vi "Replace Column Object.vi"(8 "error in (no error)":errorcluster, 10 "Column Object":refnum<class "Column Interface.lvclass">, 11 "Table in":refnum<class "Table.lvclass">) -> (0 "error out":errorcluster, 3 "Table out":refnum<class "Table.lvclass">)   [LabVIEW 2020, in "Table.lvlib" / "Table.lvclass"]
uses:
  Table.lvclass
  Column Interface/Column Interface Class/Column Interface.lvclass
  Table.lvclass/Table.ctl
  <vilib>/Utility/miscctls.llb/LVMapReplaceAction.ctl
  Table Configuration Interface/Table Configuration Interface.lvclass
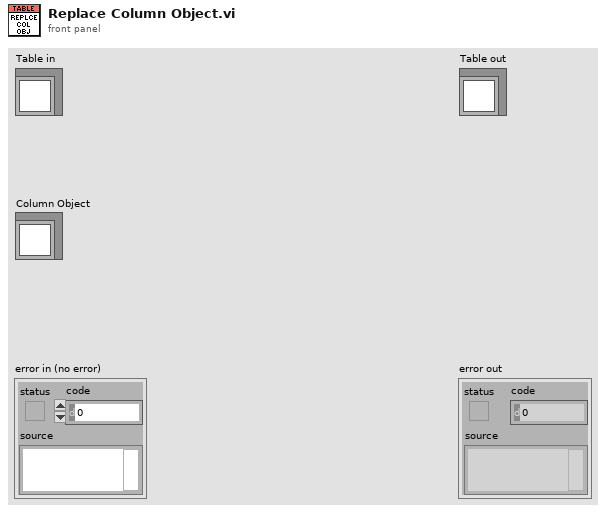
[diagram p1: front panel]
types:
  T1 = typedef "LVMapReplaceAction.ctl" = enum32{"Modify Entry only if found", "Add or Modify Entry", "Delete Entry"}
  T2 = map{string, refnum<class "Column Interface.lvclass">}
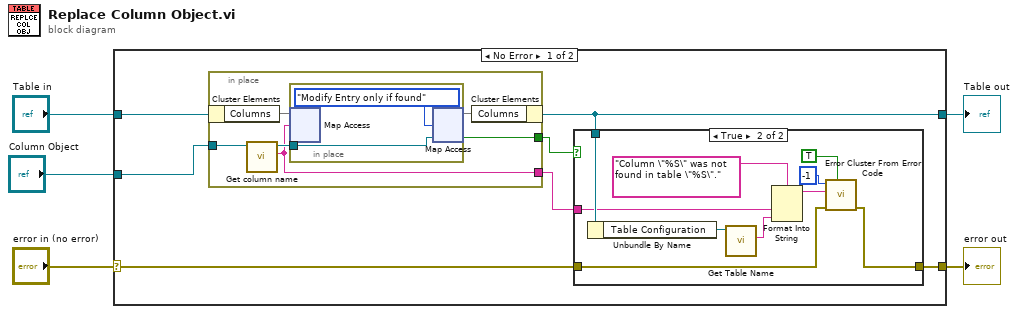
[diagram p0: block diagram]
diagram:
  n1 = case shown="No Error" "error in (no error)" {
    selector: "error in (no error)" -> [w6 w33]
    tunnel: [w7 w33] -> w4
    tunnel: [w10 w32] -> w2
    tunnel: "Table in" -> [w12 w32]
    tunnel: "Column Object" -> [w11 _]
    frame No Error {
      n2 = in-place {
        in-place-border: w11 -> [w29]
        in-place-border: [w25] -> w9
        in-place-border: [w24] -> w8
        n3 = in-place-cluster #1(w12) -> ("Columns"=w28:T2)
        n4 = call-dynamic "Get column name.vi"("Column Interface in"=w29) -> ("Name"=w24:string, "Column Interface out"=w27:refnum<class "Column Interface.lvclass">)  [unwired: 8 in, 1 out]
        n5 = in-place {
          in-place-border: w27 -> [w30]
          n6 = in-place-map #2(w28, w24) -> ()  [unwired: 1 in, 2 out]
          n7 = in-place-map #2(w30, LVMapReplaceAction."Modify Entry only if found" ("action")) -> (w26:T2, w25:bool)  [unwired: 1 out]
        }
        n8 = in-place-cluster #1("Columns"=w26) -> (w10:refnum<class "Table.lvclass">)
      }
      n9 = case shown="True" w9 {
        tunnel: w10 -> [_ w22]
        tunnel: w8 -> [_ w20]
        tunnel: [w13 w15] -> w7
        tunnel: w6 -> [w13 w14]
        frame False {
        }
        frame True {
          n10 = Unbundle By Name(w22) -> ("Table Configuration"=w21:refnum<class "Table Configuration Interface.lvclass">)
          n11 = call-dynamic "Get Table Name.vi"("Table Configuration Interface in"=w21) -> ("Table Name"=w19:string)  [unwired: 8 in, 2 out]
          n12 = Format Into String(format string="Column \"%S\" was not found in table \"%S\".", w20, w19) -> (resulting string=w18:string)  [unwired: 2 in, 1 out]
          n13 = call <vilib>:"Error Cluster From Error Code.vi"("show call chain? (False)"=TRUE, "error in (no error)"=w14, "error message (\"\")"=w18, "error code (0)"=-1) -> ("error out"=w15:errorcluster)  [unwired: 5 in]
        }
      }
    }
    frame Error {
    }
  }
  "error out" <- w4
  "Table out" <- w2
